vi "Read subject.vi"(8 "error in (no error)":errorcluster, 11 "TimeStamper in":refnum<class "TimeStamper.lvclass">) -> (0 "error out":errorcluster, 2 "subject":string, 3 "TimeStamper out":refnum<class "TimeStamper.lvclass">)   [LabVIEW 2014, in "TimeStamper.lvclass"]
uses:
  TimeStamper.lvclass
  TimeStamper.lvclass/TimeStamper.ctl
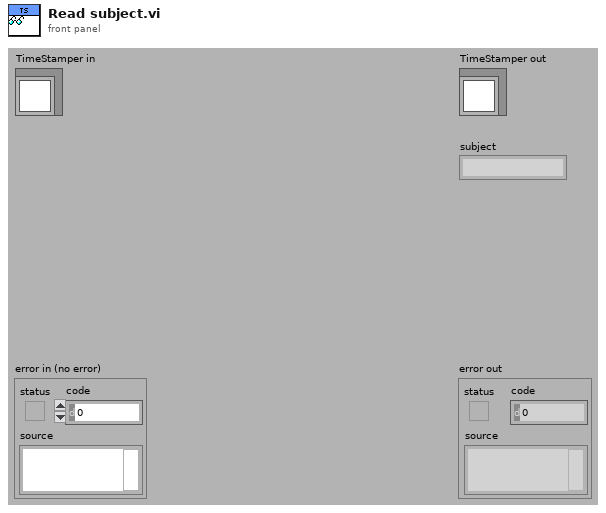
[diagram p1: front panel]
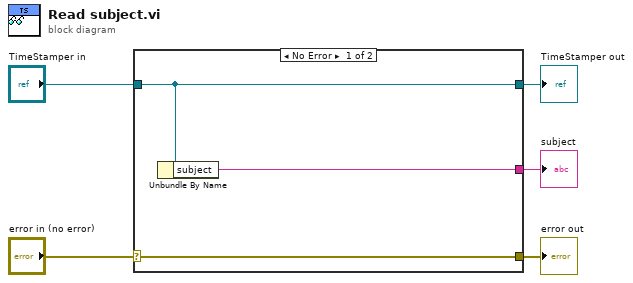
[diagram p0: block diagram]
diagram:
  n1 = case shown="No Error" "error in (no error)" {
    selector: "error in (no error)" -> [w8 w9]
    tunnel: [w8 w9] -> w4
    tunnel: [w7 w10] -> w2
    tunnel: "TimeStamper in" -> [w7 w10]
    tunnel: [w6 _] -> w1
    frame No Error {
      n2 = Unbundle By Name(w7) -> ("subject"=w6:string)
    }
    frame Error {
    }
  }
  "error out" <- w4
  "TimeStamper out" <- w2
  "subject" <- w1
